vi "nosilec_LabVIEW.vi"() -> ()   [LabVIEW 2018]
panel:
  out "Faza":dynamicdata(graph) caption="Phase"
  out "Magnituda":dynamicdata(graph) caption="Magnitude"
  out "data":dynamicdata(graph)
  out "Kladivo [N]":dynamicdata(graph)
  out "Pospeškomer [g]":dynamicdata(graph)
  in  "Enable":bool=TRUE
  in  "Filename":path=path "C:/Users/Bizjan/Desktop/Fakulteta/4. SEMESTER/Nihanja struktur/Nosilec/Meritve/udarec.lvm"
  in  "stop (F)":bool
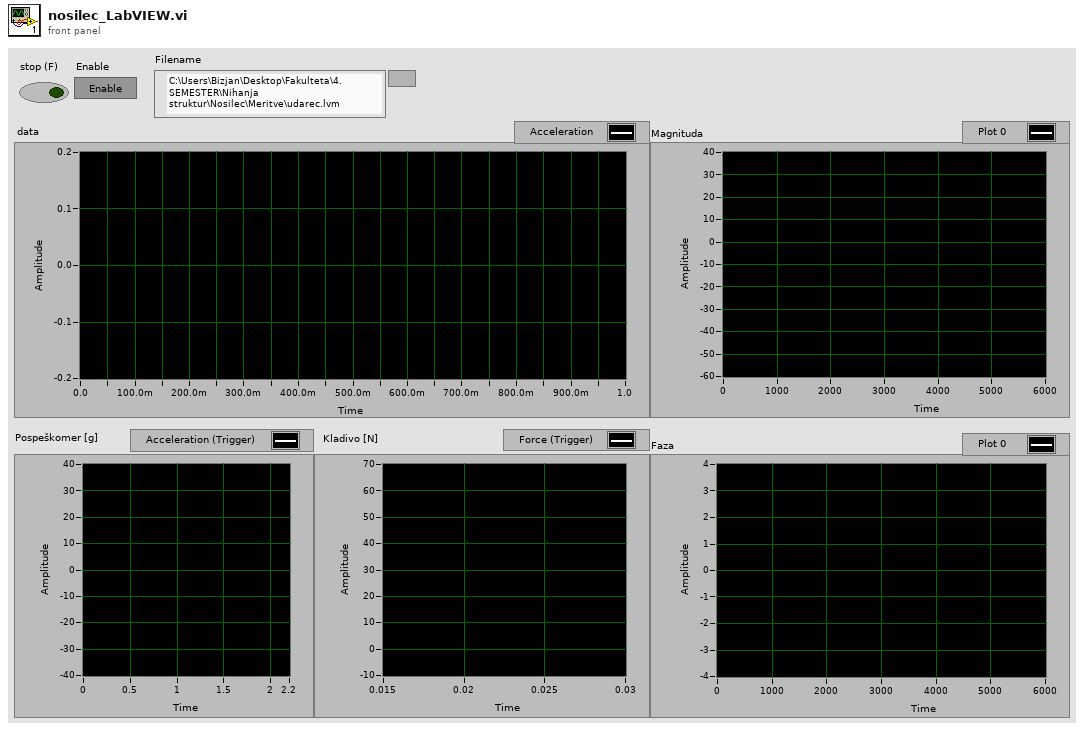
[diagram p1: front panel]
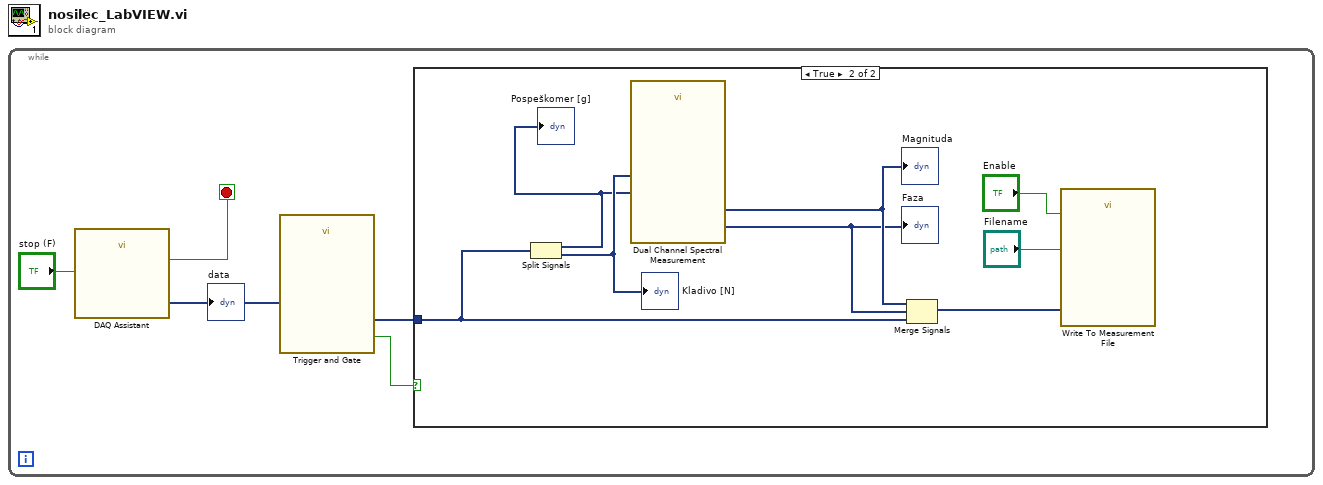
[diagram p0: block diagram]
diagram:
  n1 = while {
    stop <- w4 stop-if-true
    n2 = call "DAQ Assistant"("stop (F)"="stop (F)") -> ("data"=w1:dynamicdata, "stopped"=w4:bool)  [unwired: 15 in, 2 out]
    "data" <- w1
    n3 = call "Trigger and Gate"("Signals"=w1) -> ("Triggered Signals"=w3:dynamicdata, "Data Available"=w2:bool)  [unwired: 7 in, 2 out]
    n4 = case shown="True" w2 {
      tunnel: w3 -> [_ w11]
      frame False {
      }
      frame True {
        n5 = Split Signals(w11) -> (w6:dynamicdata, w7:dynamicdata)  [unwired: 2 in]
        "Pospeškomer [g]" <- w6
        "Kladivo [N]" <- w7
        n6 = call "Dual Channel Spectral Measurement"("Input Signal B"=w6, "Input Signal A"=w7) -> ("Phase"=w8:dynamicdata, "Magnitude"=w9:dynamicdata)  [unwired: 7 in, 1 out]
        "Magnituda" <- w9
        "Faza" <- w8
        n7 = Merge Signals(w9, w8, w11) -> (w10:dynamicdata)
        n8 = call "Write To Measurement File"("Signals"=w10, "Enable"="Enable", "Filename"="Filename") -> ()  [unwired: 14 in, 3 out]
      }
    }
  }
